vi "Tickbox - Untick.vi"(8 "Error In":errorcluster, 11 "Tickbox Ref":refnum<vi>) -> (0 "Error Out":errorcluster)   [LabVIEW 2022 SP3]
doc: "<add documentation here>"
panel:
  # "Development\nControls or indicators that are useful for development or testing, but which are not outputs of the VI."
  # "Input\nInputs to the VI"
  # "Output\nOutputs of the VI"
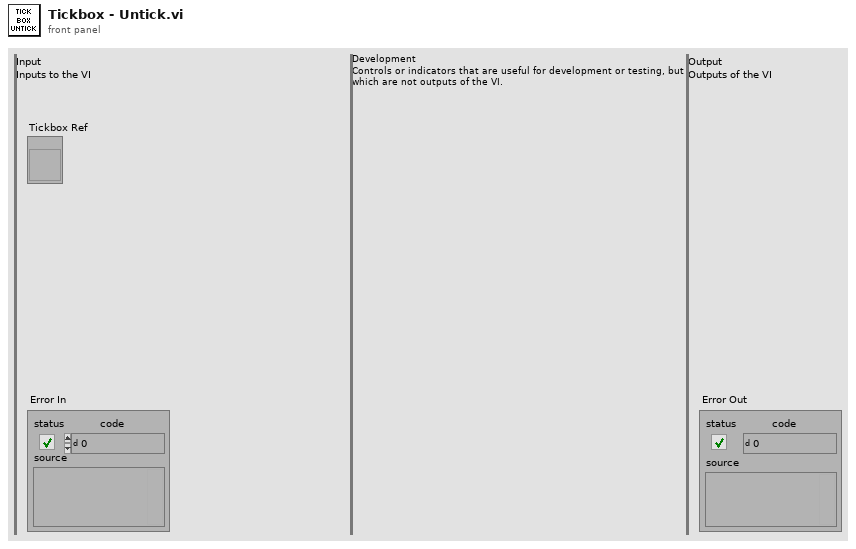
[diagram p1: front panel]
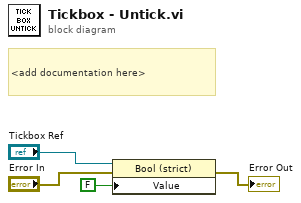
[diagram p0: block diagram]
diagram:
  # "<add documentation here>"
  n1 = property class="Bool (strict)"(reference="Tickbox Ref", error in="Error In", "Value"=FALSE) -> (error out=→"Error Out":errorcluster)  [unwired: 1 out]
